vi "MeasAction.vi"(8 "error in (no error)":errorcluster caption="entrée d'erreur (pas d'erreur)", 9 "CurvePointIndex":i32, 10 "AllPointIndex":i32, 11 "InstrClassIn":refnum<class "AttoAMC300.lvclass"> caption="DNL_LabVIEW Object in") -> (0 "error out":errorcluster caption="sortie d'erreur", 2 "MeasDatOut":dbl[](array[numeric]), 3 "InstrClassOut":refnum<class "AttoAMC300.lvclass"> caption="DNL_LabVIEW Object out")   [LabVIEW 2019, in "AttoAMC300.lvclass"]
uses:
  AttoAMC300.lvclass
  AttoAMC300.lvclass/AttoAMC300.ctl
  <userlib>/AMC300/AMC_VIs.lvlib
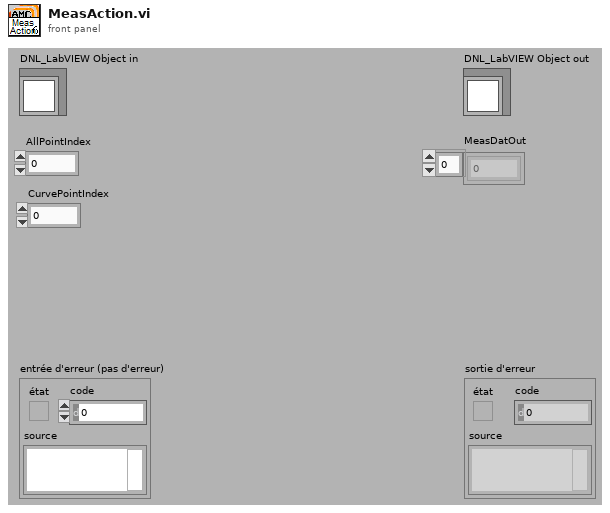
[diagram p1: front panel]
types:
  T1 = typedef "AttoAMC300.lvclass/AttoAMC300_Func.ctl" = enum16{"Position (um)", "MotionMon (um)"}
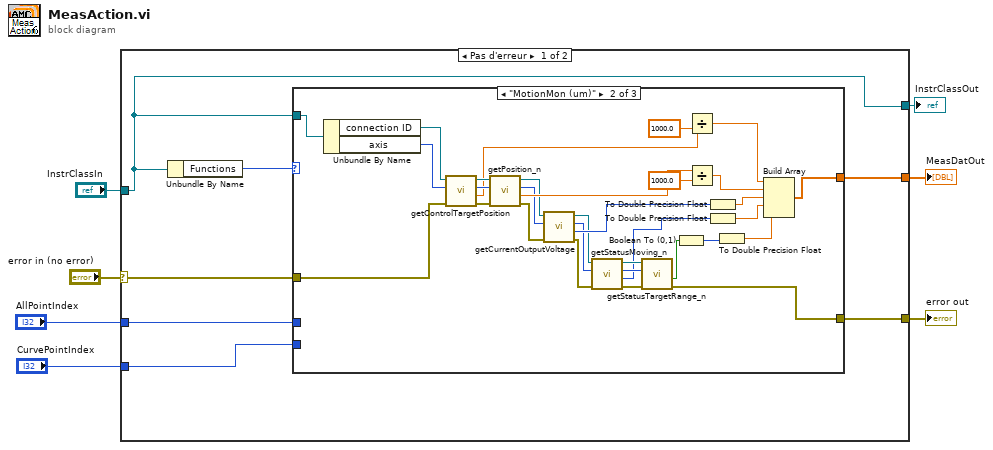
[diagram p0: block diagram]
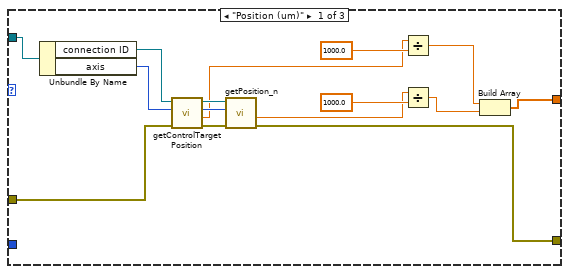
[diagram p2: hidden frame]
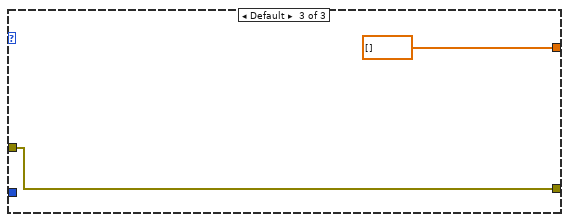
[diagram p3: hidden frame]
diagram:
  n1 = case shown="Pas d'erreur" "error in (no error)" {
    selector: "error in (no error)" -> [w10 w63]
    tunnel: "InstrClassIn" -> [w8 w64]
    tunnel: [w8 w64] -> w5
    tunnel: "AllPointIndex" -> [w14 _]
    tunnel: [w13 w63] -> w3
    tunnel: [w12 _] -> w2
    tunnel: "CurvePointIndex" -> [w9 _]
    frame No Error {
      n2 = Unbundle By Name(w8) -> ("Functions"=w11:T1)
      n3 = case shown="\"MotionMon (um)\"" w11 {
        tunnel: w14 -> [_ _ _]
        tunnel: [w15 w35 w62] -> w13
        tunnel: [w28 w59 dbl[] [] ("Outputs")] -> w12
        tunnel: w10 -> [w23 w54 w62]
        tunnel: w9 -> [_ _ _]
        tunnel: w8 -> [w29 w60 _]
        frame "Position (um)" {
          n4 = Unbundle By Name(w29) -> ("connection ID"=w22:refnum<k5>, "axis"=w21:i32)
          n5 = call <userlib>:"getControlTargetPosition.vi"("error in"=w23, "axis"=w21, "connection ID"=w22) -> ("error out"=w24:errorcluster, "position [nm/µdeg]"=w17:dbl, "axis_out"=w19:i32, "connection ID"=w20:refnum<k5>)  [unwired: 5 in]
          n6 = call <userlib>:"getPosition_n.vi"("error in"=w24, "axis"=w19, "connection ID"=w20) -> ("error out"=w15:errorcluster, "position"=w26:dbl)  [unwired: 5 in, 2 out]
          n7 = Divide(x=w17, y=1000.0) -> (x/y=w16:dbl)
          n8 = Divide(x=w26, y=1000.0) -> (x/y=w25:dbl)
          n9 = Build Array(w16, w25) -> (w28:dbl[])
        }
        frame "MotionMon (um)" {
          n10 = Unbundle By Name(w60) -> ("connection ID"=w53:refnum<k5>, "axis"=w52:i32)
          n11 = call <userlib>:"getControlTargetPosition.vi"("error in"=w54, "axis"=w52, "connection ID"=w53) -> ("error out"=w55:errorcluster, "position [nm/µdeg]"=w48:dbl, "axis_out"=w50:i32, "connection ID"=w51:refnum<k5>)  [unwired: 5 in]
          n12 = call <userlib>:"getPosition_n.vi"("error in"=w55, "axis"=w50, "connection ID"=w51) -> ("error out"=w46:errorcluster, "position"=w57:dbl, "axis_out"=w42:i32, "connection ID"=w43:refnum<k5>)  [unwired: 5 in]
          n13 = call <userlib>:"getCurrentOutputVoltage.vi"("error in"=w46, "axis"=w42, "connection ID"=w43) -> ("error out"=w40:errorcluster, "amplitude"=w44:i32, "axis_out"=w39:i32, "connection ID"=w41:refnum<k5>)  [unwired: 5 in]
          n14 = call <userlib>:"getStatusMoving_n.vi"("error in"=w40, "axis"=w39, "connection ID"=w41) -> ("error out"=w36:errorcluster, "status"=w34:i32, "axis_out"=w38:i32, "connection ID"=w37:refnum<k5>)  [unwired: 5 in]
          n15 = call <userlib>:"getStatusTargetRange_n.vi"("error in"=w36, "axis"=w38, "connection ID"=w37) -> ("error out"=w35:errorcluster, "in_range"=w30:bool)  [unwired: 5 in, 2 out]
          n16 = Boolean To (0,1)(Boolean=w30) -> (0, 1=w32:i16)
          n17 = Divide(x=w48, y=1000.0) -> (x/y=w47:dbl)
          n18 = Divide(x=w57, y=1000.0) -> (x/y=w56:dbl)
          n19 = To Double Precision Float(number=w44) -> (double precision float=w45:dbl)
          n20 = To Double Precision Float(number=w34) -> (double precision float=w33:dbl)
          n21 = To Double Precision Float(number=w32) -> (double precision float=w31:dbl)
          n22 = Build Array(w47, w56, w45, w33, w31) -> (w59:dbl[])
        }
        frame Default {
        }
      }
    }
    frame Error {
    }
  }
  "error out" <- w3
  "InstrClassOut" <- w5
  "MeasDatOut" <- w2
